vi "test_libssh2_channel_free.vi"() -> ()   [LabVIEW 2013, in "libssh2_integration_tests.lvlib"]
uses:
  libssh2_integration_tests.lvlib
  <vilib>/addons/_JKI Toolkits/Caraya/classes/Test/Test.lvclass
  support/support.lvlib
  libssh2/libssh2.lvlib
  <vilib>/addons/_JKI Toolkits/Caraya/classes/Assert/Assert.lvclass
panel:
  out "error out":errorcluster
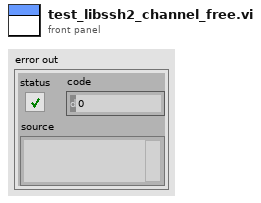
[diagram p1: front panel]
types:
  T1 = typedef "libssh2.lvlib/Session Refnum.ctl" = refnum<k1>
  T2 = typedef "libssh2.lvlib/Channel Refnum.ctl" = refnum<k1>
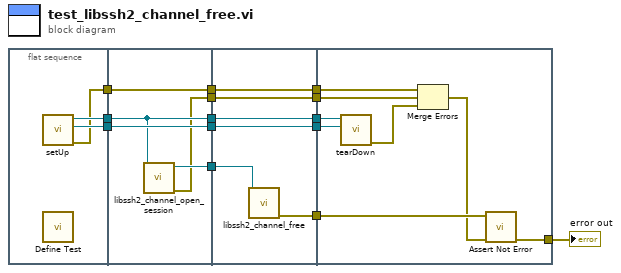
[diagram p0: block diagram]
diagram:
  n1 = flat-sequence {
    tunnel: [w17] -> w14
    tunnel: [w16] -> w13
    tunnel: [w15] -> w7
    tunnel: w14 -> [w21]
    tunnel: w13 -> [w22]
    tunnel: [w21] -> w5
    tunnel: [w22] -> w4
    tunnel: [w20] -> w3
    tunnel: w7 -> [w19]
    tunnel: [w19] -> w2
    tunnel: [w18] -> w1
    tunnel: w5 -> [w28]
    tunnel: w4 -> [w27]
    tunnel: w3 -> [w26]
    tunnel: [w28] -> w12
    tunnel: [w27] -> w11
    tunnel: [w23] -> w10
    tunnel: [w25] -> w8
    tunnel: w2 -> [w24]
    tunnel: [w24] -> w6
    tunnel: w1 -> [w25]
    tunnel: w12 -> [w35]
    tunnel: w11 -> [w34]
    tunnel: w10 -> [w36]
    tunnel: [w33] -> w9
    tunnel: w8 -> [w31]
    tunnel: w6 -> [w30]
    frame #0 {
      n2 = call "setUp.vi"() -> ("error out"=w15:errorcluster, "connection ID"=w16:refnum<k5>, "session"=w17:T1)  [unwired: 9 in]
      n3 = call <vilib>:"Define Test.vi"() -> ()  [unwired: 10 in, 2 out]
    }
    frame #1 {
      n4 = call "libssh2_channel_open_session.vi"("session"=w21) -> ("error out"=w18:errorcluster, "channel"=w20:T2)  [unwired: 9 in]
    }
    frame #2 {
      n5 = call "libssh2_channel_free.vi"("channel"=w26) -> ("error out"=w23:errorcluster)  [unwired: 10 in]
    }
    frame #3 {
      n6 = call "tearDown.vi"("connection ID"=w34, "session"=w35) -> ("error out"=w32:errorcluster)  [unwired: 9 in]
      n7 = Merge Errors(w30, w31, w32) -> (w29:errorcluster)
      n8 = call <vilib>:"Assert Not Error.vi"("error in (no error)"=w29, "Not Error?"=w36) -> ("error out"=w33:errorcluster)  [unwired: 8 in, 1 out]
    }
  }
  "error out" <- w9
